vi "FlexRIO5761.vi"() -> ()   [LabVIEW 2013]
uses:
  Control 1.ctl
  <vilib>/Platform/TimedLoop/XDataNode/timing_clust.ctl
  <vilib>/Platform/TimedLoop/XDataNode/nitl_modes.ctl
  <vilib>/Platform/TimedLoop/XDataNode/wakeup.ctl
  vis5761/libs/ctl/AcquisitionStateControl.ctl
  vis5761/libs/ctl/SelectedChannels.ctl
  <vilib>/rvi/DataTransferAndStorage/Container/Common/niFpgaContainerExecOnDevCompGetState.vi
  <vilib>/rvi/FIFO/Fifo_Resource/nirvififoEmulationClearFpgaImpl.vi
  <vilib>/rvi/DataTransferAndStorage/Container/Common/niFpgaContainerGetUniqueNameForEmu.vi
  <vilib>/rvi/interface/RandomDataEmulation/nirviRandomDataFPGAFIFO.vi
  <vilib>/rvi/interface/RandomDataEmulation/niFpgaRandomDataHandleErrors.vi
  <vilib>/rvi/eio/common/nirviEmuReportErrorAndStop.vi
  <vilib>/rvi/Emulation/niFpgaSctlEmulationGetInTimedLoop.vi
  <vilib>/rvi/Emulation/niFpgaEmulationReportErrorSimple.vi
  <vilib>/rvi/Emulation/niFpgaGetClockAttributes.vi
  <vilib>/rvi/eio/common/nirviEmuTemplateMethod_errors.vi
  <vilib>/rvi/Emulation/niFpgaCriticalErrorInLSC.vi
  <vilib>/rvi/FIFO/Fifo_Resource/nirvififoEmulationGetNumberOfElementsToReadFpgaImpl.vi
  <vilib>/rvi/FIFO/Fifo_Resource/nirvififoEmulationReadFpgaImpl.vi
  <vilib>/rvi/FIFO/Fifo_Resource/nirvififoEmulationWriteFpgaImpl.vi
  vis5761/libs/common/GlobalReg.vi
  <vilib>/rvi/Emulation/niFpgaProcessEmulError.vi
  <vilib>/Platform/TimedLoop/XDataNode/XDataNode.xnode
  <vilib>/rvi/DataTransferAndStorage/Container/XNode/niFpgaContainer.xnode
  <vilib>/rvi/FIFO/Fifo_Resource/niFpgaFifoEmulationRefIn.vi
  <vilib>/eio/EIONode/EIONode.xnode
  <vilib>/rvi/FIFO/Fifo_Resource/nirvififoEmulationClear.vi
  <vilib>/rvi/interface/RandomDataEmulation/nirviRandomDataFpgaReadWriteTemplate.vi
  <vilib>/Platform/TimedLoop/XDataNode/XDNodeRunTimeDep.lvlib
  vis5761/libs/IRIO.lvlib
panel:
  in  "DMA Control":T1={"DMATtoHOSTNCh"=[4], "DMATtoHOSTFrameType"=[0], "DMATtoHOSTSampleSize"=[2], "DMATtoHOSTBlockNWords"=[4096]}
  in  "Tab Control":T2(tab)=enum."Data Acquisition"
  out "Platform":enum8{"FlexRIO", "cRIO", "RSeries"}(ring)
  out "FPGAVIversion":u8[](array[numeric])=[1, 1]
  out "InitDone":bool
  out "RIOAdapterCorrect":bool
  out "Fref":u32=125000000
  out "DevQualityStatus":u8
  out "DevTemp":i16=-10244
  out "DevProfile":u8 format="%x"
  in  "DAQStartStop":bool
  in  "DebugMode":bool
  out "Expected IO Module ID":u32 format="%x"
  out "InsertedIOModule ID":u32
  out "DMATtoHOSTNCh":T3[](array[typedef])=[4]
  out "DMATtoHOSTFrameType":u8[](array[numeric])
  out "DMATtoHOSTSampleSize":u8[](array[numeric])=[2]
  out "DMATtoHOSTBlockNWords":u16[](array[numeric])=[4096]
  in  "DMATtoHOSTSamplingRate0":u16=10000
  in  "DMATtoHOSTEnable0":bool
  out "DMATtoHOSTOverflows":u16
  out "auxAI5":i32
  out "auxAI4":i32
  out "auxAI3":i32
  out "auxAI2":i32
  out "auxAI1":i32
  out "auxAI0":i32
  in  "auxAO5":i32
  in  "auxAO4":i32
  in  "auxAO3":i32
  in  "auxAO2":i32
  in  "auxAO1":i32
  in  "auxAO0":i32
  out "auxDI5":bool
  out "auxDI4":bool
  out "auxDI3":bool
  out "auxDI2":bool
  out "auxDI1":bool
  out "auxDI0":bool
  in  "auxDO3":bool
  in  "auxDO4":bool
  in  "auxDO5":bool
  in  "auxDO2":bool
  in  "auxDO1":bool
  in  "auxDO0":bool
  in  "SGUpdateRate0":u32=40
  in  "SGPhase0":u32
  in  "SGFreq0":u32=100000
  in  "SGAmp0":u16
  in  "AO0":i32
  out "auxAI9":i32
  out "SGNo":u8=2 format="%x"
  out "auxAI10":i32
  in  "SGSignalType1":u8
  in  "SGAmp1":u16
  in  "SGPhase1":u32
  in  "SGFreq1":u32=100000
  in  "SGUpdateRate1":u32=40
  in  "AO1":i32
  in  "AOEnable1":bool
  out "SGFref0":u32=100000000
  out "SGFref1":u32=100000000
  in  "AOEnable0":bool
  in  "SGSignalType0":u8
  # "Inputs"
  # "Aux \nDigital Inputs"
  # "Aux \nAnalog Inputs"
  # "Digital Inputs"
  # "Outputs"
  # "Number of WF gen"
  # "Analog Outputs"
  # "Aux Digital \nOutput"
  # "Digital\nOutputs"
  # "Aux Analog \nOutput"
  # "Signal Generator 1"
  # "Signal Generator 0"
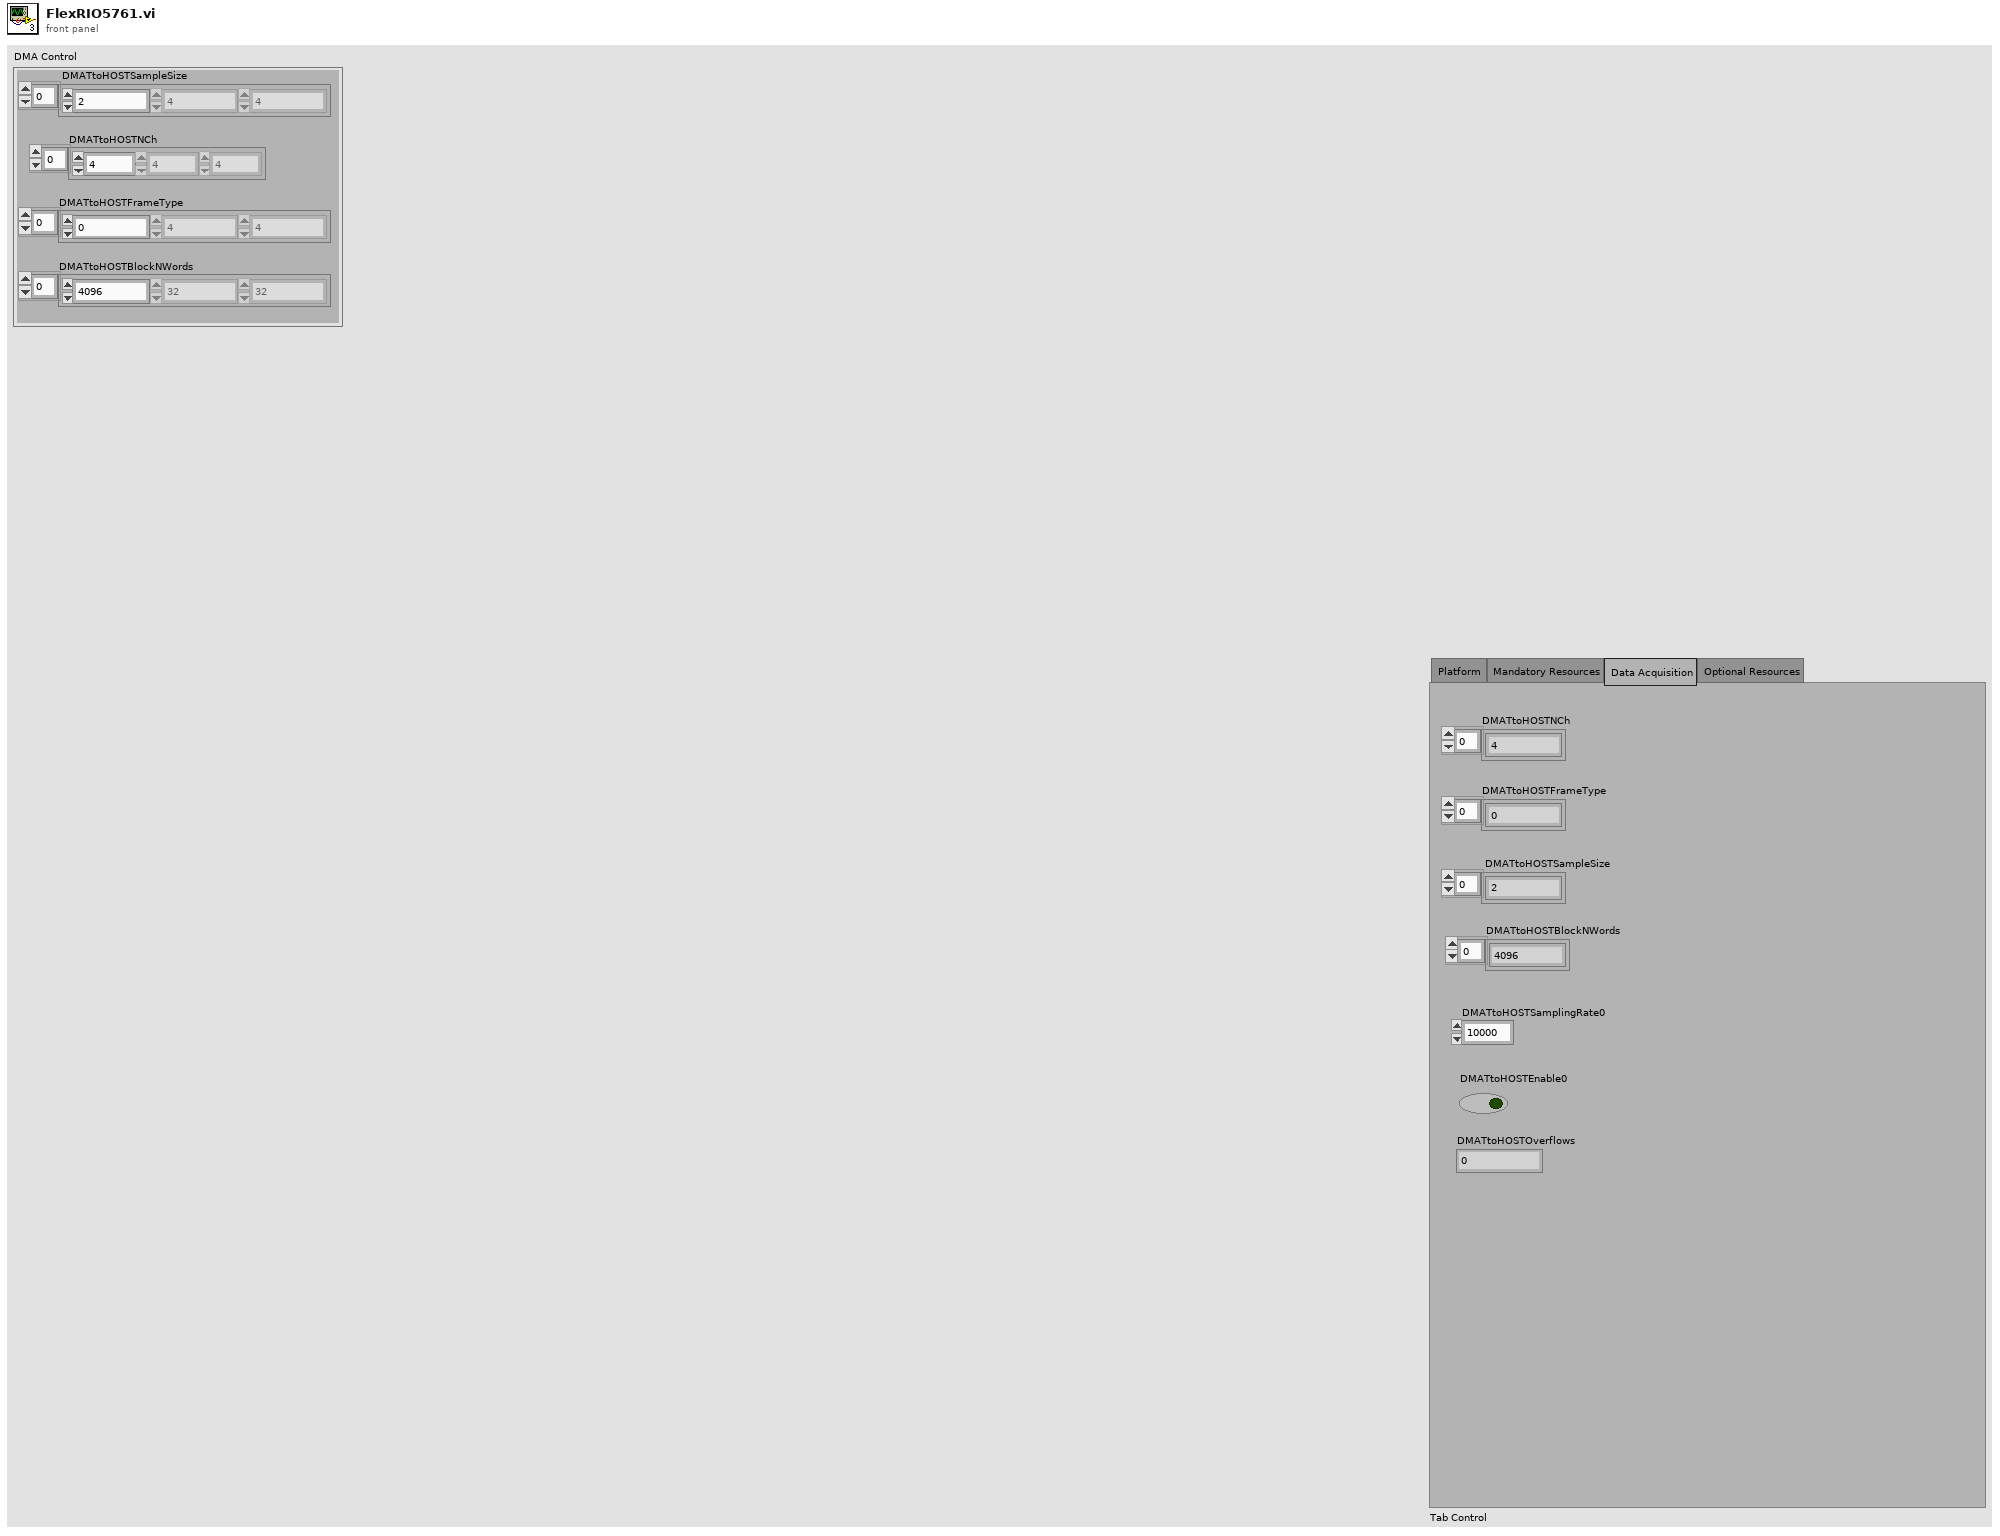
[diagram p1: front panel]
types:
  T1 = cluster{"DMATtoHOSTNCh":u16[], "DMATtoHOSTFrameType":u8[], "DMATtoHOSTSampleSize":u8[], "DMATtoHOSTBlockNWords":u16[]}
  T2 = enum32{"Platform", "Mandatory Resources", "Data Acquisition", "Optional Resources"}
  T3 = typedef "Control 1.ctl" = u16
  T4 = typedef "XDNodeRunTimeDep.lvlib/timing_clust.ctl" = cluster{"Expected End [f-1]":u64, "Actual End [f-1]":u64, "Finished Late? [f-1]":bool, "Expected End [i-1]":u64, "Actual End [i-1]":u64, "Finished Late? [i-1]":bool, "Expected Start [i]":u64, "Actual Start [i]":u64, "Expected Start [f]":u64, "Actual Start [f]":u64, "Source Name":string, "Structure Name":string, "Period":i64, "Deadline":i64, "Offset":i64, "Start":i64, "Priority":i32, "Timeout":i32, "Mode":T5, "Wakeup Reason":T6, "Error":errorcluster, "Source Type":string, "Secondary Source Type":string, "Global End Time":u64, "Global Start Time":u64, "Frame Duration":u64, "Iteration Duration":u64, "Assigned CPU":i32, "I/O Scan Engine Mode":u32}
  T5 = typedef "XDNodeRunTimeDep.lvlib/nitl_modes.ctl" = enum32{"No Change", "Process missed periods, maintain original phase", "Discard missed periods, maintain original phase", "Process missed periods, ignore original phase", "Discard missed periods, ignore original phase"}
  T6 = typedef "XDNodeRunTimeDep.lvlib/wakeup.ctl" = enum32{"Normal", "Aborted", "Asynchronous wakeup", "Timing source error", "Timed loop error", "Timeout"}
  T7 = typedef "IRIO.lvlib/AcquisitionStateControl.ctl" = enum16{"Idle", "Acq"}
  T8 = typedef "IRIO.lvlib/SelectedChannels.ctl" = enum16{"Empty", "AI0", "AI1", "AI2", "AI3", "SignalGenerator0", "SignalGenerator1", "DDCA_PORT0", "DDCA_PORT1", "DDCA_PORT2", "DDCB_PORT0", "DDCB_PORT1", "DDCB_PORT2"}
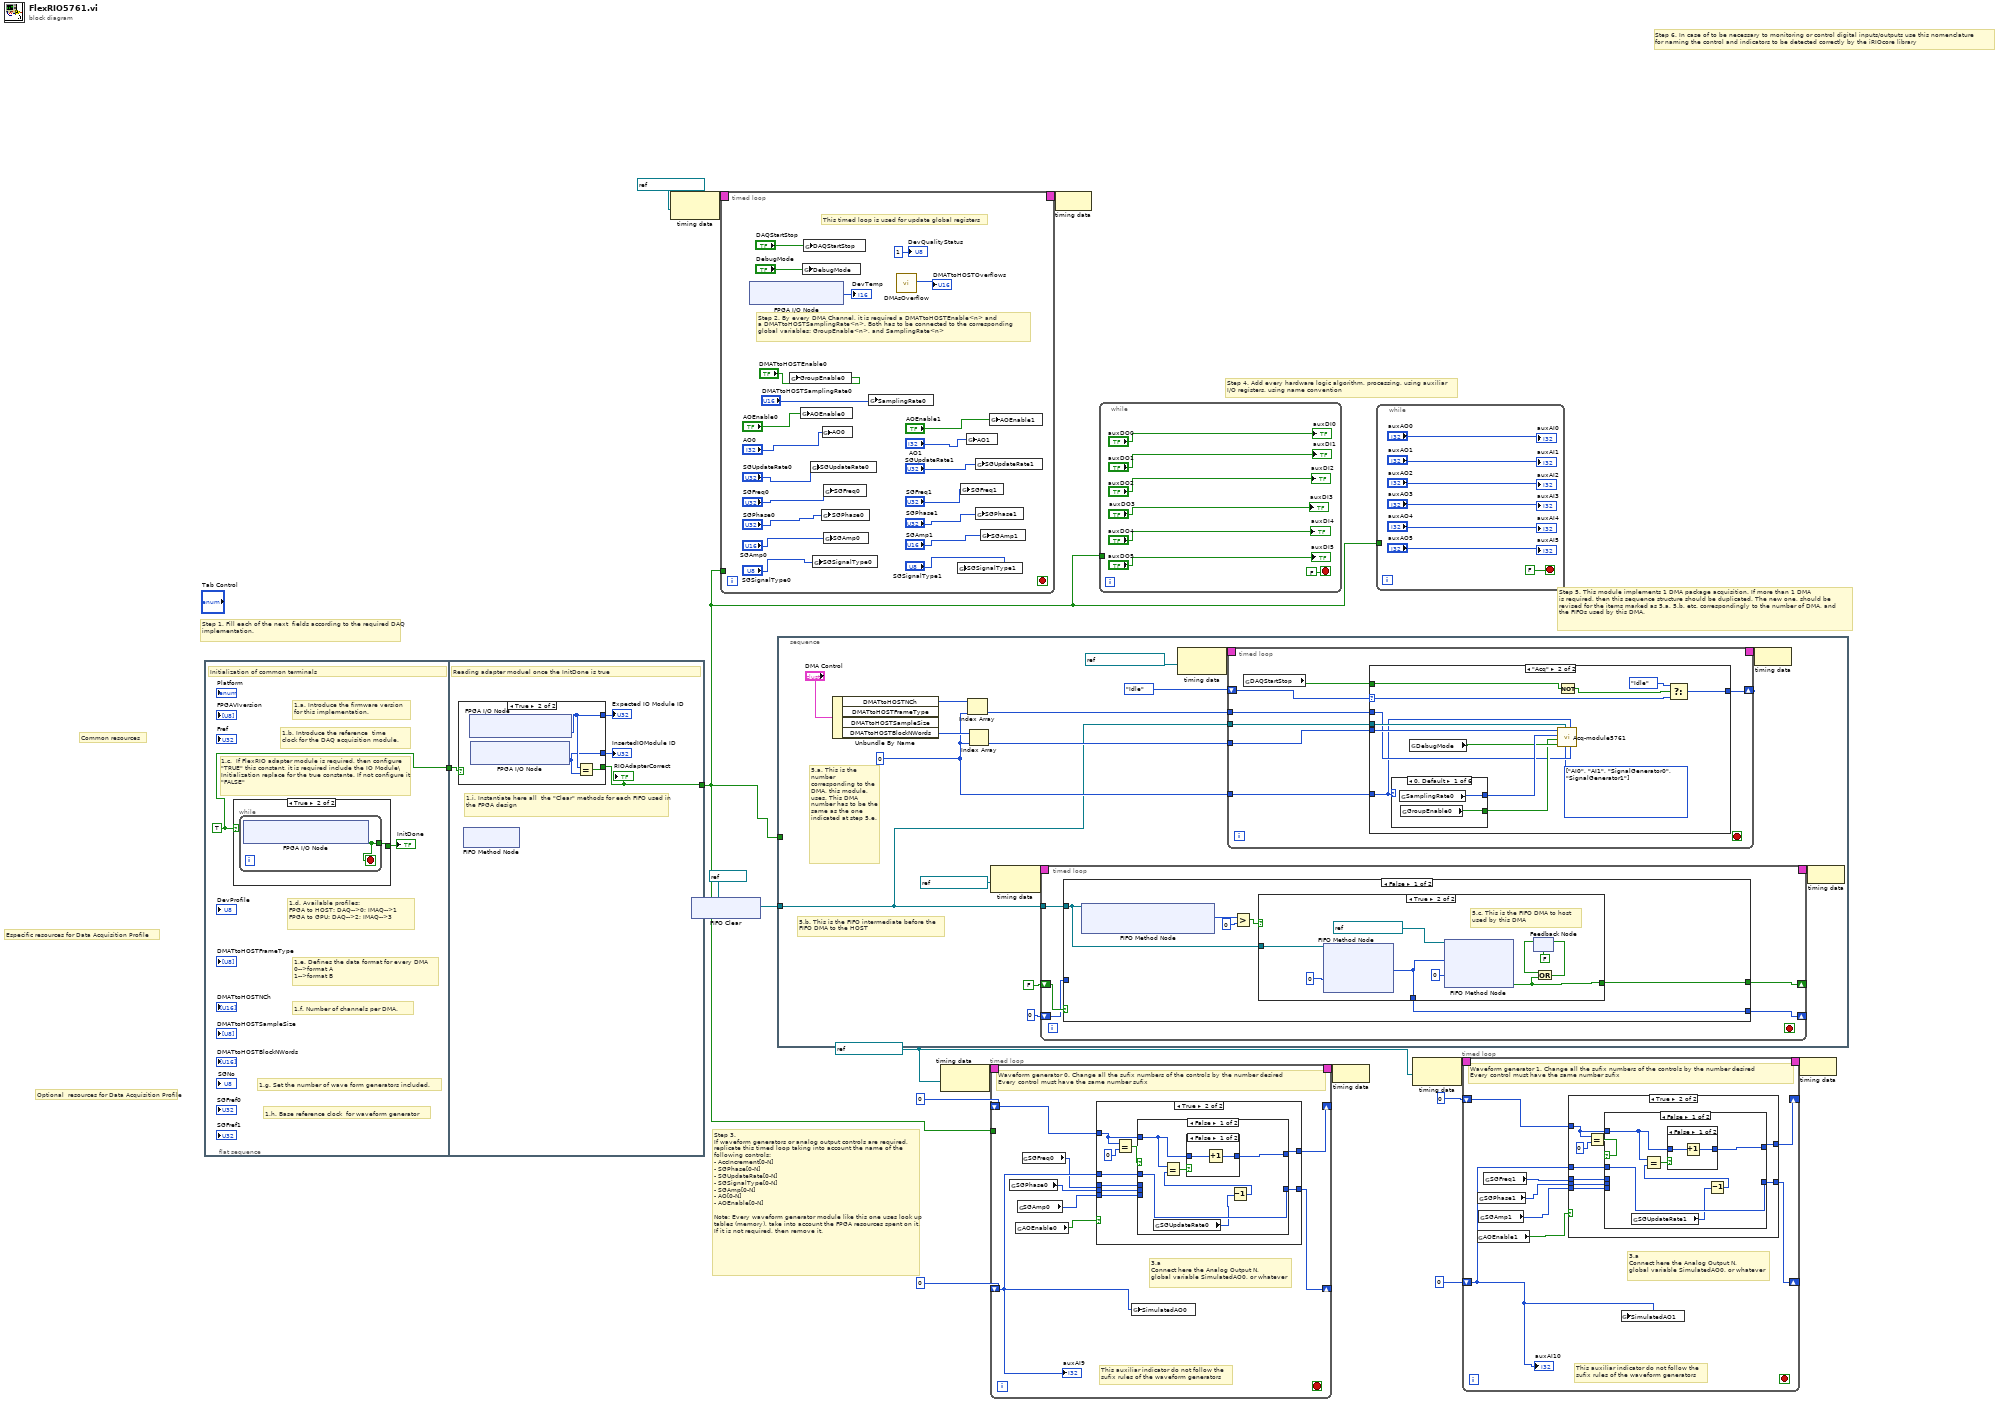
[diagram p0: block diagram]
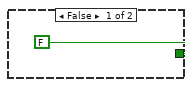
[diagram p2: hidden frame]
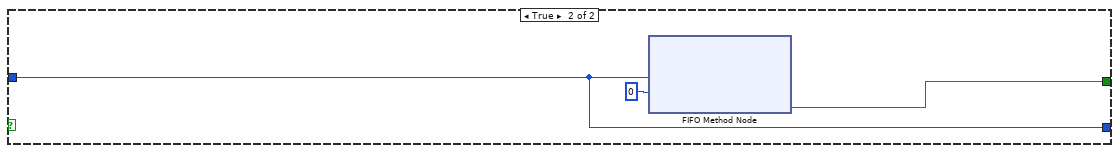
[diagram p3: hidden frame]
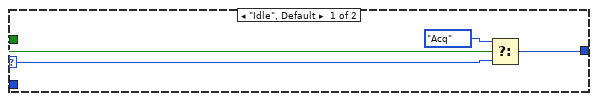
[diagram p4: hidden frame]
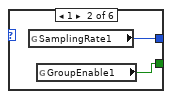
[diagram p5: hidden frame]
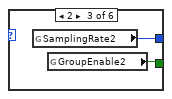
[diagram p6: hidden frame]
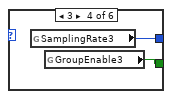
[diagram p7: hidden frame]
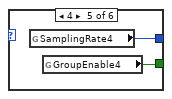
[diagram p8: hidden frame]
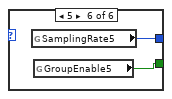
[diagram p9: hidden frame]
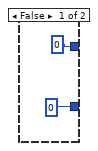
[diagram p10: hidden frame]
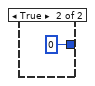
[diagram p11: hidden frame]
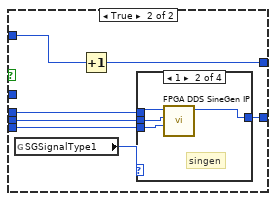
[diagram p12: hidden frame]
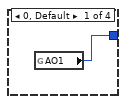
[diagram p13: hidden frame]
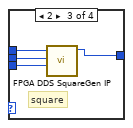
[diagram p14: hidden frame]
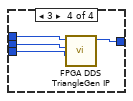
[diagram p15: hidden frame]
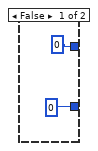
[diagram p16: hidden frame]
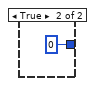
[diagram p17: hidden frame]
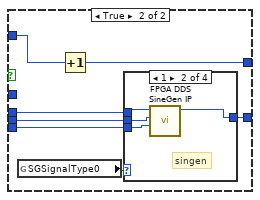
[diagram p18: hidden frame]
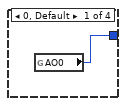
[diagram p19: hidden frame]
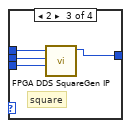
[diagram p20: hidden frame]
diagram:
  w4 = refnum<k21> "100 MHz Clock" ("Source Name")
  # "Step 5. This module implements 1 DMA package acquisition. If more than 1 DMA \nis required, then this sequence structure should be duplicated. The new one, should be \nrevised for the items marked as 5.a, 5.b, etc. correspondingly to the number of DMA, and \nthe FIFOs used by this DMA."
  # "Step 3.\nIf waveform generators or analog output controls are required,\nreplicate this timed loop taking into account the name of the \nfollowing controls:\n- AccIncrement[0-N]\n- SGPhase[0-N]\n- SGUpdateRate[0-N]\n- SGSignalType[0-N]\n- SGAmp[0-N]\n- AO[0-N]\n- AOEnable[0-N]\n\nNote: Every waveform generator module like this one uses look up tables (memory), take into account the FPGA resources spent on it.  If it is not required, then remove it."
  # "Step 6. In case of to be necessary to monitoring or control digital inputs/outputs use this nomenclature\nfor naming the control and indicators to be detected correctly by the iRIOcore library"
  # "Optional  resources for Data Acquisition Profile"
  # "Especific resources for Data Acquisition Profile"
  # "Common resources"
  # "Step 4. Add every hardware logic algorithm, processing, using auxiliar \nI/O registers, using name convention"
  # "Step 1. Fill each of the next  fields according to the required DAQ implementation."
  n1 = flat-sequence {
    tunnel: [w17] -> w16
    tunnel: [w24] -> w1
    tunnel: w16 -> [w23]
    frame #0 {
      w17 = TRUE
      # "1.h. Base reference clock  for waveform generator"
      # "1.g. Set the number of wave form generators included."
      # "1.e. Defines the data format for every DMA\n0-->format A\n1-->format B"
      # "1.c.  If FlexRIO adapter module is required, then configure \"TRUE\" this constant, it is required include the IO Module\\Initialization replace for the true constante. If not configure it \"FALSE\""
      # "1.a. Introduce the firmware version \nfor this implementation."
      # "1.b. Introduce the reference  time \nclock for the DAQ acquisition module."
      # "1.f. Number of channels per DMA."
      # "1.d. Available profiles: \nFPGA to HOST: DAQ-->0; IMAQ-->1\nFPGA to GPU: DAQ-->2; IMAQ-->3"
      # "Initialization of common terminals"
      n2 = case shown="True" w17 {
        tunnel: [w19 w21] -> w18
        frame False {
          n3 = while {
            tunnel: [w20] -> w19
            stop <- w20 stop-if-true
            w20 = TRUE
          }
        }
        frame True {
          n4 = while {
            tunnel: [w22] -> w21
            stop <- w22 stop-if-true
            n5 = xnode "FPGA I/O Node"() -> ("IO Module\\Initialization Done"=w22:bool)  [unwired: 1 in, 1 out]
          }
        }
      }
      "InitDone" <- w18
    }
    frame #1 {
      # "1.i. Instantiate here all  the \"Clear\" methods for each FIFO used in the FPGA design"
      # "Reading adapter moduel once the InitDone is true"
      n6 = case shown="True" w23 {
        tunnel: [TRUE w31] -> w24
        tunnel: [w28 w30] -> w26
        tunnel: [w28 w29] -> w25
        frame False {
          w28 = u32 0
        }
        frame True {
          n7 = xnode "FPGA I/O Node"() -> ("Expected IO Module ID"=w30:u32)  [unwired: 1 in, 1 out]
          n8 = xnode "FPGA I/O Node"() -> ("Inserted IO Module ID"=w29:u32)  [unwired: 1 in, 1 out]
          n9 = Equal?(x=w30, y=w29) -> (x = y?=w31:bool)
        }
      }
      "Expected IO Module ID" <- w26
      "InsertedIOModule ID" <- w25
      "RIOAdapterCorrect" <- w24
      n10 = xnode ("FIFO Method Node")() -> ()  [unwired: 1 in, 1 out]
    }
  }
  n11 = node-c288(refnum<k21> "100 MHz Clock" ("Source Name")) -> (w11:T4)
  n12 = xnode ("FIFO Clear")("FIFO In"=refnum<k21> "FIFO0" ("IntermediateFIFO")) -> ("FIFO Out"=w2:refnum<k21>)
  n13 = timed-loop {
    timing: w11 -> [_]
    timing-out: [_] -> w10
    tunnel: w1 -> [_]
    stop <- _ stop-if-true
    # "This timed loop is used for update global registers"
    # "Step 2. By every DMA Channel, it is required a DMATtoHOSTEnable<n> and\na DMATtoHOSTSamplingRate<n>. Both has to be connected to the corresponding\nglobal variables: GroupEnable<n>, and SamplingRate<n>"
    n14 = xnode "FPGA I/O Node"() -> ("Device Temperature"=→"DevTemp":i16)  [unwired: 1 in, 1 out]
    n15 = global write "GlobalReg.vi" "GroupEnable0"("DMATtoHOSTEnable0") -> ()
    n16 = global write "GlobalReg.vi" "AOEnable0"("AOEnable0") -> ()
    n17 = global write "GlobalReg.vi" "DebugMode"("DebugMode") -> ()
    n18 = global write "GlobalReg.vi" "DAQStartStop"("DAQStartStop") -> ()
    n19 = global write "GlobalReg.vi" "SGUpdateRate0"("SGUpdateRate0") -> ()
    n20 = global write "GlobalReg.vi" "SGSignalType0"("SGSignalType0") -> ()
    n21 = global write "GlobalReg.vi" "SGPhase0"("SGPhase0") -> ()
    n22 = global write "GlobalReg.vi" "AO0"("AO0") -> ()
    n23 = global write "GlobalReg.vi" "SGAmp0"("SGAmp0") -> ()
    n24 = global write "GlobalReg.vi" "SGFreq0"("SGFreq0") -> ()
    n25 = global write "GlobalReg.vi" "SamplingRate0"("DMATtoHOSTSamplingRate0") -> ()
    n26 = call "DMAsOverflow.vi"() -> ("DMAsOverFlow"=→"DMATtoHOSTOverflows":u16)  [unwired: 11 in]
    n27 = global write "GlobalReg.vi" "SGSignalType1"("SGSignalType1") -> ()
    n28 = global write "GlobalReg.vi" "SGFreq1"("SGFreq1") -> ()
    n29 = global write "GlobalReg.vi" "AO1"("AO1") -> ()
    n30 = global write "GlobalReg.vi" "SGUpdateRate1"("SGUpdateRate1") -> ()
    n31 = global write "GlobalReg.vi" "SGPhase1"("SGPhase1") -> ()
    n32 = global write "GlobalReg.vi" "SGAmp1"("SGAmp1") -> ()
    n33 = global write "GlobalReg.vi" "AOEnable1"("AOEnable1") -> ()
    "DevQualityStatus" <- u8 1 ("DevQualityStatus")
  }
  n34 = stacked-sequence {
    tunnel: w2 -> [w55]
    tunnel: w1 -> [_]
    frame #0 {
      w57 = 0 ("DMA number")
      # "5.b. This is the FIFO intermediate before the \nFIFO DMA to the HOST"
      # "5.a. This is the number corresponding to the \nDMA, this module, uses. This DMA \nnumber has to be the same as the one indicated at step 5.e."
      n35 = Unbundle By Name("DMA Control") -> ("DMATtoHOSTNCh"=w61:u16[], "DMATtoHOSTBlockNWords"=w63:u16[])  [unwired: 2 out]
      n36 = Index Array(array=w61, index=w57) -> (element=w60:u16)
      n37 = Index Array(array=w63, index=w57) -> (element=w62:u16)
      n38 = node-c288(refnum<k21> "100 MHz Clock" ("Base Clock")) -> (w68:T4)
      n39 = timed-loop {
        timing: w68 -> [_]
        timing-out: [_] -> w67
        shift-right: [w75] -> _
        shift-left: FALSE ("Timed Out?") -> [w74]
        shift-right: [w73] -> _
        shift-left: u64 0 -> [w72]
        tunnel: w55 -> [w71]
        stop <- _ stop-if-true
        n40 = case shown="False" w74 {
          tunnel: [w78 w93] -> w75
          tunnel: [w77 w92] -> w73
          tunnel: w72 -> [_ w92]
          tunnel: w71 -> [w76 _]
          frame False {
            n41 = xnode ("FIFO Method Node")("FIFO In"=w76) -> ("Number of Elements to Read"=w81:u32)  [unwired: 1 out]
            n42 = Greater?(x=w81, y=u32 0) -> (0:w79:bool)
            n43 = case shown="True" w79 {
              tunnel: [FALSE ("Timed Out?") w88] -> w78
              tunnel: [_ w89] -> w77
              tunnel: w76 -> [_ w84]
              frame False {
              }
              frame True {
                # "5.c. This is the FIFO DMA to host \nused by this DMA"
                n44 = xnode ("FIFO Method Node")("Timeout"=0, "FIFO In"=w84) -> ("Element"=w89:u64)  [unwired: 2 out]
                n45 = xnode ("FIFO Method Node")("Element"=w89, "Timeout"=0, "FIFO In"=refnum<k21> "DMATtoHOST0" ("DMATtoHOSTFIFO")) -> ("Timed Out?"=w88:bool)  [unwired: 1 out]
                n46 = feedback #1(FALSE) -> (w87:bool)
                n47 = Or(x=w87, y=w88) -> (x .or. y?=w86:bool)
                n48 = feedback-in #1(w86) -> ()
              }
            }
          }
          frame True {
            n49 = xnode ("FIFO Method Node")("Element"=w92, "Timeout"=0) -> ("Timed Out?"=w93:bool)  [unwired: 1 in, 1 out]
          }
        }
      }
      n50 = node-c288(refnum<k21> "IO Module Clock 0" ("Module Clock")) -> (w70:T4)
      n51 = timed-loop {
        timing: w70 -> [_]
        timing-out: [_] -> w69
        shift-right: [w107] -> _
        shift-left: AcquisitionStateControl."Idle" ("Enum") -> [w102]
        tunnel: w57 -> [w105]
        tunnel: w60 -> [w104]
        tunnel: w55 -> [w103]
        tunnel: w62 -> [w101]
        stop <- _ stop-if-true
        n52 = global read "GlobalReg.vi" "DAQStartStop"() -> (w106:bool)
        n53 = case shown="\"Acq\"" w102 {
          selector: w102 -> [w109 w123]
          tunnel: w106 -> [w111 w120]
          tunnel: [w108 w122] -> w107
          tunnel: w105 -> [_ w113]
          tunnel: w104 -> [_ w114]
          tunnel: w103 -> [_ w119]
          tunnel: w101 -> [_ w115]
          frame "Idle", Default {
            n54 = Select(t=AcquisitionStateControl."Acq" ("Enum"), s=w111, f=w109) -> (s? t:f=w108:T7)
          }
          frame "Acq" {
            w112 = T8[] [enum."AI0", enum."AI1", enum."SignalGenerator0", enum."SignalGenerator1"] items=["Empty", "AI0", "AI1", "AI2", "AI3", "SignalGenerator0", "SignalGenerator1", "DDCA_PORT0", "DDCA_PORT1", "DDCA_PORT2", "DDCB_PORT0", "DDCB_PORT1", "DDCB_PORT2"] ("Selected Channels")
            n55 = case shown="0, Default" w113 {
              tunnel: [w126 w128 w130 w132 w134 w136] -> w118
              tunnel: [w125 w127 w129 w131 w133 w135] -> w116
              frame 0, Default {
                n56 = global read "GlobalReg.vi" "SamplingRate0"() -> (w126:u16)
                n57 = global read "GlobalReg.vi" "GroupEnable0"() -> (w125:bool)
              }
              frame 1 {
                n58 = global read "GlobalReg.vi" "SamplingRate1"() -> (w128:u16)
                n59 = global read "GlobalReg.vi" "GroupEnable1"() -> (w127:bool)
              }
              frame 2 {
                n60 = global read "GlobalReg.vi" "SamplingRate2"() -> (w130:u16)
                n61 = global read "GlobalReg.vi" "GroupEnable2"() -> (w129:bool)
              }
              frame 3 {
                n62 = global read "GlobalReg.vi" "SamplingRate3"() -> (w132:u16)
                n63 = global read "GlobalReg.vi" "GroupEnable3"() -> (w131:bool)
              }
              frame 4 {
                n64 = global read "GlobalReg.vi" "SamplingRate4"() -> (w134:u16)
                n65 = global read "GlobalReg.vi" "GroupEnable4"() -> (w133:bool)
              }
              frame 5 {
                n66 = global read "GlobalReg.vi" "SamplingRate5"() -> (w136:u16)
                n67 = global read "GlobalReg.vi" "GroupEnable5"() -> (w135:bool)
              }
            }
            n68 = global read "GlobalReg.vi" "DebugMode"() -> (w117:bool)
            n69 = call "Acq-module5761.vi"("NumChannels"=w114, "DMA number"=w113, "Selected Channels"=w112, "IntermediateFIFO"=w119, "DebugActivation"=w117, "GroupEnableN"=w116, "SamplingRateN(DecimationFactor)"=w118, "DMATtoHOSTBlockNWords"=w115) -> ()  [unwired: 4 in]
            n70 = Not(x=w120) -> (.not. x?=w121:bool)
            n71 = Select(t=AcquisitionStateControl."Idle" ("Enum"), s=w121, f=w123) -> (s? t:f=w122:T7)
          }
        }
      }
      n72 = node-c288(w69) -> ()
      n73 = node-c288(w67) -> ()
    }
  }
  n74 = node-c288(w4) -> (w15:T4)
  n75 = timed-loop {
    shift-right: [w150] -> _
    shift-left: i16 0 ("Signal Value") -> [w147]
    timing: w15 -> [_]
    timing-out: [_] -> w14
    shift-right: [w148] -> _
    shift-left: u32 0 -> [w149]
    tunnel: w1 -> [_]
    stop <- _ stop-if-true
    # "This auxiliar indicator do not follow the \nsufix rules of the waveform generators"
    # "3.a\nConnect here the Analog Output N,\nglobal variable SimulatedAO0, or whatever"
    # "Waveform generator 0. Change all the sufix numbers of the controls by the number desired\nEvery control must have the same number sufix"
    n76 = global read "GlobalReg.vi" "SGPhase0"() -> (w145:u32)
    n77 = global read "GlobalReg.vi" "AOEnable0"() -> (w143:bool)
    n78 = global read "GlobalReg.vi" "SGAmp0"() -> (w144:u16)
    n79 = global read "GlobalReg.vi" "SGFreq0"() -> (w146:u32)
    n80 = case shown="True" w143 {
      tunnel: w146 -> [_ w161]
      tunnel: w145 -> [_ w160]
      tunnel: w144 -> [_ w159]
      tunnel: [i16 0 w158] -> w150
      tunnel: w149 -> [_ w155]
      tunnel: [u32 0 w154] -> w148
      tunnel: w147 -> [_ w153]
      frame False {
      }
      frame True {
        n81 = Equal?(x=w155, y=u32 0) -> (x = y?=w157:bool)
        n82 = case shown="False" w157 {
          tunnel: w161 -> [_ w177]
          tunnel: w160 -> [_ w176]
          tunnel: w159 -> [_ w175]
          tunnel: [w166 w174] -> w158
          tunnel: w155 -> [w165 w173]
          tunnel: [w167 w172] -> w154
          tunnel: w153 -> [w166 _]
          frame False {
            n83 = global read "GlobalReg.vi" "SGUpdateRate0"() -> (w162:u32)
            n84 = Decrement(x=w162) -> (x-1=w163:u32)
            n85 = Equal?(x=w165, y=w163) -> (x = y?=w164:bool)
            n86 = case shown="False" w164 {
              tunnel: w165 -> [w169 _]
              tunnel: [w168 u32 0] -> w167
              frame False {
                n87 = Increment(x=w169) -> (x+1=w168:u32)
              }
              frame True {
              }
            }
          }
          frame True {
            n88 = global read "GlobalReg.vi" "SGSignalType0"() -> (w171:u8)
            n89 = Increment(x=w173) -> (x+1=w172:u32)
            n90 = case shown="1" w171 {
              tunnel: w177 -> [_ w182 w186 w190]
              tunnel: w176 -> [_ w181 w185 w189]
              tunnel: w175 -> [_ w180 w184 w188]
              tunnel: [w178 w179 w183 w187] -> w174
              frame 0, Default {
                n91 = global read "GlobalReg.vi" "AO0"() -> (w178:i32)
              }
              frame 1 {
                # "singen"
                n92 = call "FPGA DDS SineGen IP.vi"("Signal Amplitude (x 2^15)"=w180, "Phase Shift"=w181, "Accumulator Increment"=w182) -> ("Signal Value"=w179:i16)  [unwired: 7 in, 1 out]
              }
              frame 2 {
                # "square"
                n93 = call "FPGA DDS SquareGen IP.vi"("Signal Amplitude (x 2^15)"=w184, "Phase Shift"=w185, "Accumulator Increment"=w186) -> ("Signal Value"=w183:i16)  [unwired: 7 in, 1 out]
              }
              frame 3 {
                n94 = call "FPGA DDS TriangleGen IP.vi"("Signal Amplitude (x 2^15)"=w188, "Phase Shift"=w189, "Accumulator Increment"=w190) -> ("Signal Value"=w187:i16)  [unwired: 7 in, 1 out]
              }
            }
          }
        }
      }
    }
    n95 = global write "GlobalReg.vi" "SimulatedAO0"(w147) -> ()
    "auxAI9" <- w147
  }
  n96 = node-c288(w10) -> ()
  n97 = while {
    tunnel: w1 -> [_]
    stop <- FALSE stop-if-true
    "auxDI0" <- "auxDO0"
    "auxDI1" <- "auxDO1"
    "auxDI2" <- "auxDO2"
    "auxDI3" <- "auxDO3"
    "auxDI4" <- "auxDO4"
    "auxDI5" <- "auxDO5"
  }
  n98 = node-c288(w14) -> ()
  n99 = while {
    tunnel: w1 -> [_]
    stop <- FALSE stop-if-true
    "auxAI0" <- "auxAO0"
    "auxAI1" <- "auxAO1"
    "auxAI2" <- "auxAO2"
    "auxAI3" <- "auxAO3"
    "auxAI4" <- "auxAO4"
    "auxAI5" <- "auxAO5"
  }
  n100 = node-c288(w4) -> (w8:T4)
  n101 = timed-loop {
    shift-right: [w214] -> _
    shift-left: i16 0 ("Signal Value") -> [w207]
    timing: w8 -> [_]
    timing-out: [_] -> w7
    shift-right: [w212] -> _
    shift-left: u32 0 -> [w213]
    stop <- _ stop-if-true
    # "This auxiliar indicator do not follow the \nsufix rules of the waveform generators"
    # "3.a\nConnect here the Analog Output N,\nglobal variable SimulatedAO0, or whatever"
    # "Waveform generator 1. Change all the sufix numbers of the controls by the number desired\nEvery control must have the same number sufix"
    n102 = global read "GlobalReg.vi" "AOEnable1"() -> (w208:bool)
    n103 = global read "GlobalReg.vi" "SGPhase1"() -> (w210:u32)
    n104 = global read "GlobalReg.vi" "SGAmp1"() -> (w209:u16)
    n105 = global read "GlobalReg.vi" "SGFreq1"() -> (w211:u32)
    n106 = case shown="True" w208 {
      tunnel: w211 -> [_ w225]
      tunnel: w210 -> [_ w224]
      tunnel: w209 -> [_ w223]
      tunnel: [i16 0 w222] -> w214
      tunnel: w213 -> [_ w219]
      tunnel: [u32 0 w218] -> w212
      tunnel: w207 -> [_ w217]
      frame False {
      }
      frame True {
        n107 = Equal?(x=w219, y=u32 0) -> (x = y?=w221:bool)
        n108 = case shown="False" w221 {
          tunnel: w225 -> [_ w241]
          tunnel: w224 -> [_ w240]
          tunnel: w223 -> [_ w239]
          tunnel: [w230 w238] -> w222
          tunnel: w219 -> [w229 w237]
          tunnel: [w231 w236] -> w218
          tunnel: w217 -> [w230 _]
          frame False {
            n109 = global read "GlobalReg.vi" "SGUpdateRate1"() -> (w226:u32)
            n110 = Decrement(x=w226) -> (x-1=w227:u32)
            n111 = Equal?(x=w229, y=w227) -> (x = y?=w228:bool)
            n112 = case shown="False" w228 {
              tunnel: w229 -> [w233 _]
              tunnel: [w232 u32 0] -> w231
              frame False {
                n113 = Increment(x=w233) -> (x+1=w232:u32)
              }
              frame True {
              }
            }
          }
          frame True {
            n114 = global read "GlobalReg.vi" "SGSignalType1"() -> (w235:u8)
            n115 = Increment(x=w237) -> (x+1=w236:u32)
            n116 = case shown="1" w235 {
              tunnel: w241 -> [_ w246 w250 w254]
              tunnel: w240 -> [_ w245 w249 w253]
              tunnel: w239 -> [_ w244 w248 w252]
              tunnel: [w242 w243 w247 w251] -> w238
              frame 0, Default {
                n117 = global read "GlobalReg.vi" "AO1"() -> (w242:i32)
              }
              frame 1 {
                # "singen"
                n118 = call "FPGA DDS SineGen IP.vi"("Signal Amplitude (x 2^15)"=w244, "Phase Shift"=w245, "Accumulator Increment"=w246) -> ("Signal Value"=w243:i16)  [unwired: 7 in, 1 out]
              }
              frame 2 {
                # "square"
                n119 = call "FPGA DDS SquareGen IP.vi"("Signal Amplitude (x 2^15)"=w248, "Phase Shift"=w249, "Accumulator Increment"=w250) -> ("Signal Value"=w247:i16)  [unwired: 7 in, 1 out]
              }
              frame 3 {
                n120 = call "FPGA DDS TriangleGen IP.vi"("Signal Amplitude (x 2^15)"=w252, "Phase Shift"=w253, "Accumulator Increment"=w254) -> ("Signal Value"=w251:i16)  [unwired: 7 in, 1 out]
              }
            }
          }
        }
      }
    }
    n121 = global write "GlobalReg.vi" "SimulatedAO1"(w207) -> ()
    "auxAI10" <- w207
  }
  n122 = node-c288(w7) -> ()
